vi "Read Response.vi"(8 "error in (no error)":errorcluster, 11 "VisaComms in":refnum<class "VisaComms.lvclass">) -> (0 "error out":errorcluster, 2 "Response":string, 3 "VisaComms out":refnum<class "VisaComms.lvclass">, 5 "Buffer":string)   [LabVIEW 2024, in "CTI.lvlib" / "VisaComms.lvclass"]
uses:
  VisaComms.lvclass
  VisaComms.lvclass/VisaComms.ctl
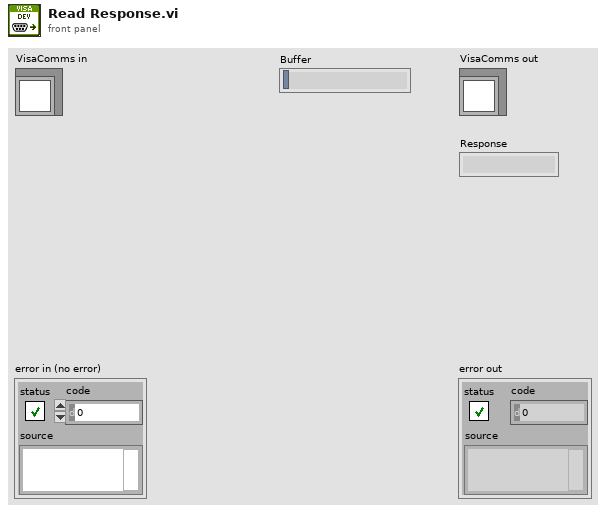
[diagram p1: front panel]
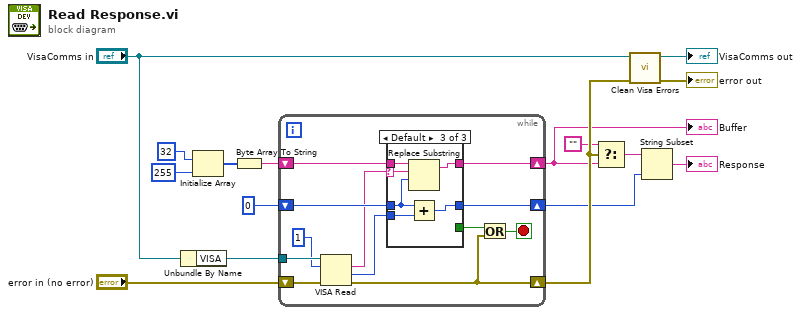
[diagram p0: block diagram]
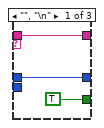
[diagram p2: hidden frame]
diagram:
  n1 = Unbundle By Name("VisaComms in") -> ("VISA"=w6:refnum<visa-resource-name>)
  n2 = Initialize Array(u8 32 ("element"), 255 ("dimension size")) -> (w13:u8[])
  n3 = Byte Array To String(unsigned byte array=w13) -> (string=w9:string)
  n4 = while {
    shift-right: [w19] -> w16
    shift-left: "error in (no error)" -> [w27]
    shift-right: [w22] -> w4
    shift-left: w9 -> [w25]
    shift-right: [w23] -> w10
    shift-left: u32 0 -> [w24]
    tunnel: w6 -> [w28]
    stop <- w20 stop-if-true
    n5 = VISA Read(VISA resource name=w28, byte count=u32 1, error in (no error)=w27) -> (read buffer=w18:string, return count=w21:u32, error out=w19:errorcluster)  [unwired: 1 out]
    n6 = case shown="Default" w18 {
      selector: w18 -> [_ _ w34]
      tunnel: w25 -> [w31 w33 w39]
      tunnel: w24 -> [w30 w32 w38]
      tunnel: [w30 w32 w37] -> w23
      tunnel: [w31 w33 w36] -> w22
      tunnel: w21 -> [_ _ w35]
      tunnel: [TRUE _ _] -> w17
      frame "", "\n" {
      }
      frame "\r" {
      }
      frame Default {
        n7 = Replace Substring(3:w38, 4:w34, 5:w39) -> (1:w36:string)  [unwired: 1 in, 1 out]
        n8 = Add(x=w38, y=w35) -> (x+y=w37:u32)
      }
    }
    n9 = Or(x=w17, y=w19) -> (x .or. y?=w20:bool)
  }
  "Buffer" <- w4
  n10 = Select(t="", s=w16, f=w4) -> (s? t:f=w11:string)
  n11 = call "Clean Visa Errors.vi"("error in (no error)"=w16, "VisaComms in"="VisaComms in") -> ("error out"=→"error out":errorcluster, "VisaComms out"=→"VisaComms out":refnum<class "VisaComms.lvclass">)  [unwired: 8 in]
  n12 = String Subset(string=w11, length (rest)=w10) -> (substring=→"Response":string)  [unwired: 1 in]
